vi "GetMultiRobotData.vi"() -> ()   [LabVIEW 2015]
uses:
  <vilib>/robotics/Simulator/NI_Robotics_Simulator.lvlib
  <instrlib>/DC Motor Controller/HAIOL/DC Motor Controller.lvclass
  RobotData.ctl
  <vilib>/robotics/Simulator/Engine/ODESimulator_Engine.lvclass
  <vilib>/robotics/Simulator/Robot Classes/Base/ODESimulator_Base_Robot.lvclass
  <vilib>/robotics/Simulator/Robot Factory/Sensor/Base/ODESimulator_Base_Sensor.lvclass
  <instrlib>/DC Motor Controller/HAIOL/Simulator/DC Motor Controller Simulator.lvclass
  <vilib>/robotics/Simulator/Engine/ctl/DeviceID.ctl
  <vilib>/robotics/Simulator/Robot Factory/Motor/ODESimulator_Motor.lvclass
  SensorType.ctl
panel:
  out "Distance":i32
  out "BUmpsize(s)":i32
  out "Array":T1[](array[typedef])
  out "SensorType":T2 items=["BumperSensor"=1, "DistanceSensor"=2, "AccelerometerSensor"=3, "Wall Sensor"=4, "Unknown"=0]
  in  "manifest file":path
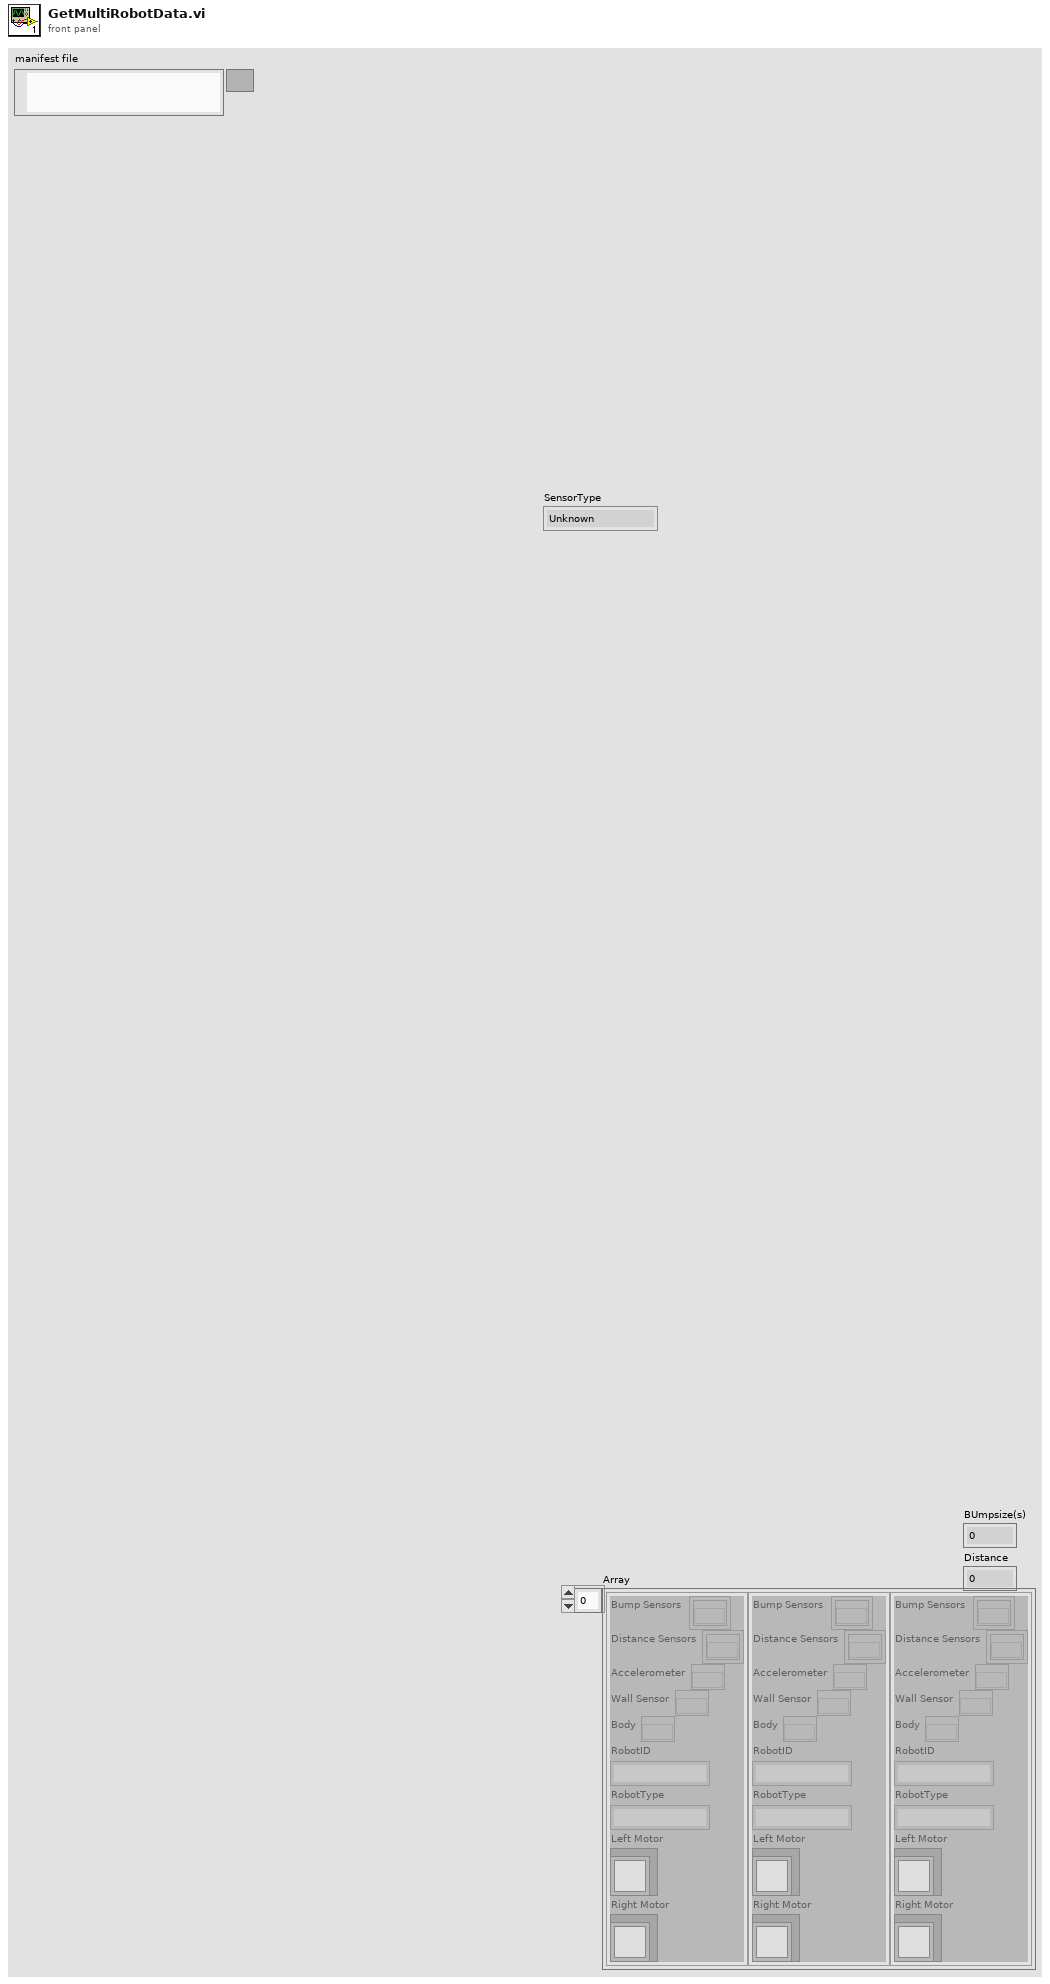
[diagram p1: front panel]
types:
  T1 = typedef "RobotData.ctl" = cluster{"Bump Sensors":refnum<k20>[], "Distance Sensors":refnum<k20>[], "Accelerometer":refnum<k20>, "Wall Sensor":refnum<k20>, "Body":refnum<k20>, "RobotID":string, "RobotType":string, "Left Motor":refnum<class "DC Motor Controller.lvclass">, "Right Motor":refnum<class "DC Motor Controller.lvclass">}
  T2 = typedef "SensorType.ctl" = u16
  T3 = typedef "RobotData.ctl" = cluster{"Bump Sensors":refnum<k20>[], "Distance Sensors":refnum<k20>[], "Accelerometer":refnum<k20>, "Wall Sensor":refnum<k20>, "Body":refnum<k20>, "RobotID":string, "Left Motor":refnum<class "DC Motor Controller.lvclass">, "Right Motor":refnum<class "DC Motor Controller.lvclass">}
  T4 = typedef "NI_Robotics_Simulator.lvlib/DeviceID.ctl" = cluster{"robot ID":string, "sensor/actuator ID":string}
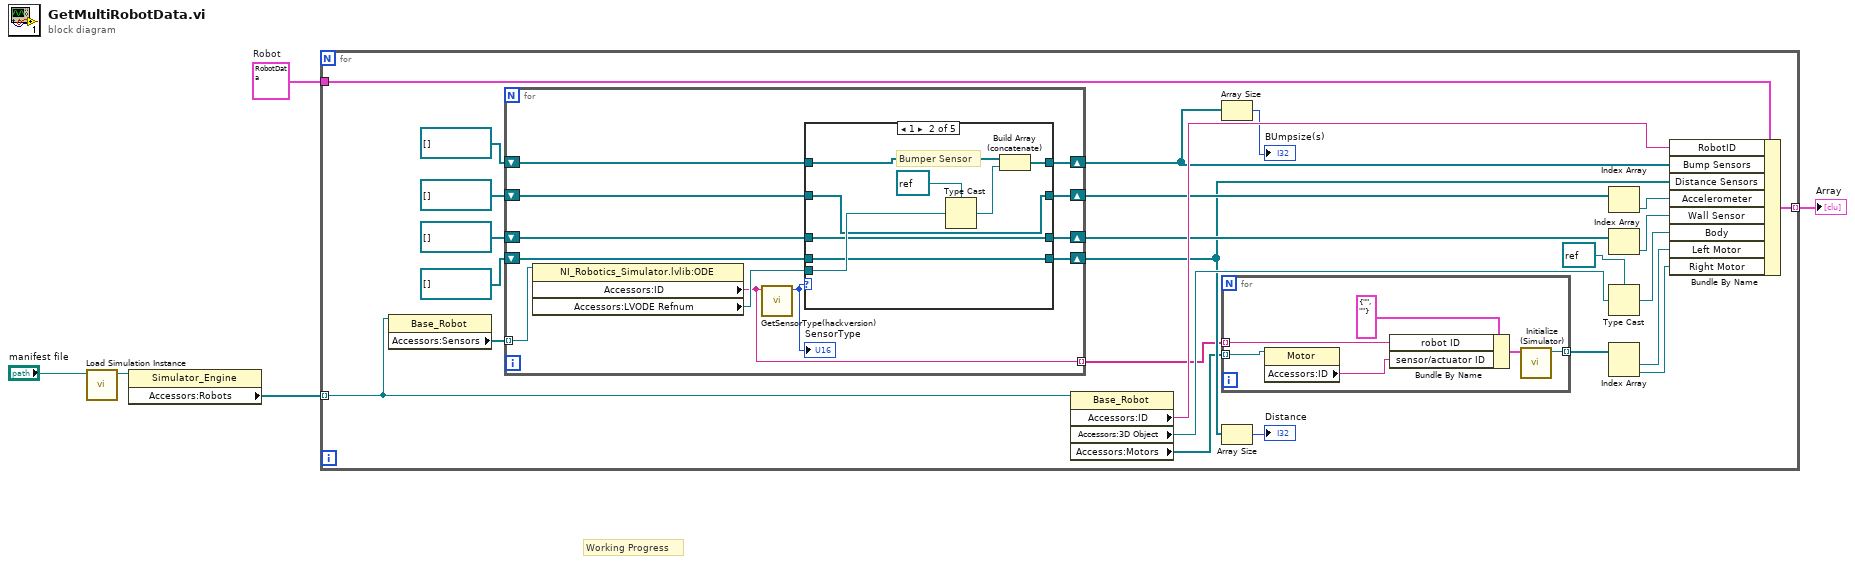
[diagram p0: block diagram]
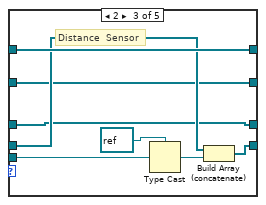
[diagram p3: hidden frame]
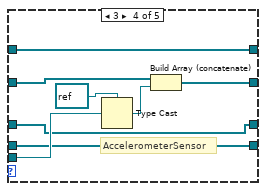
[diagram p4: hidden frame]
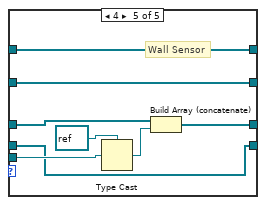
[diagram p5: hidden frame]
diagram:
  w2 = T3 {"Bump Sensors"=[], "Distance Sensors"=[], "Accelerometer"=refnum, "Wall Sensor"=refnum, "Body"=refnum, "RobotID"="", "Left Motor"=refnum, "Right Motor"=refnum}  # Robot
  # "Working Progress"
  n1 = call <vilib>:"Load Simulation Instance.vi"("manifest file"="manifest file") -> ("simulation instance"=w4:refnum<class "ODESimulator_Engine.lvclass">)  [unwired: 9 in, 1 out]
  n2 = property class="Simulator_Engine"(reference=w4) -> ("Accessors:Robots"=w3:refnum<class "ODESimulator_Base_Robot.lvclass">[])  [unwired: 1 in, 2 out]
  n3 = for {
    tunnel: w3 -> [w30] mode=indexing
    tunnel: w2 -> [w28]
    tunnel: [w15] -> w1 mode=indexing
    n4 = property class="Base_Robot"(reference=w30) -> ("Accessors:Sensors"=w29:refnum<class "ODESimulator_Base_Sensor.lvclass">[])  [unwired: 1 in, 2 out]
    n5 = for {
      tunnel: w29 -> [w48] mode=indexing
      shift-right: [w44] -> w14
      shift-left: refnum<k20>[] [] ("Bump Sensors") -> [w45]
      shift-right: [w42] -> w12
      shift-left: refnum<k20>[] [] ("Distance Sensors") -> [w43]
      shift-right: [w40] -> w22
      shift-left: refnum<k20>[] [] ("Bump Sensors") -> [w41]
      shift-right: [w38] -> w20
      shift-left: refnum<k20>[] [] ("Bump Sensors") -> [w39]
      tunnel: [w37] -> w9 mode=indexing
      n6 = property class="NI_Robotics_Simulator.lvlib:ODE"(reference=w48) -> ("Accessors:ID"=w37:string, "Accessors:LVODE Refnum"=w47:refnum<k20>)  [unwired: 1 in, 2 out]
      n7 = call "GetSensorType(hackversion).vi"("Accessors:ID"=w37) -> ("SensorType"=w46:T2)  [unwired: 9 in, 1 out]
      "SensorType" <- w46
      n8 = case shown="1" w46 {
        tunnel: w47 -> [_ w59 w67 w75 w83]
        tunnel: [w52 w57 w65 w74 w82] -> w44
        tunnel: w45 -> [w52 w56 w65 w74 w82]
        tunnel: [w51 w55 w66 w73 w81] -> w42
        tunnel: w43 -> [w51 w55 w64 w73 w81]
        tunnel: [w50 w54 w62 w70 w77] -> w40
        tunnel: w41 -> [w50 w54 w62 w72 w77]
        tunnel: w39 -> [w49 w53 w61 w69 w79]
        tunnel: [w49 w53 w61 w69 w78] -> w38
        frame 0, Default {
        }
        frame 1 {
          # "Bumper Sensor"
          n9 = Type Cast(type=refnum<k20> refnum ("LVODE Refnum"), x=w59) -> (*(type *) &x=w58:refnum<k20>)
          n10 = Build Array (concatenate)(w56, w58) -> (w57:refnum<k20>[])
        }
        frame 2 {
          # "Distance  Sensor"
          n11 = Type Cast(type=refnum<k20> refnum ("LVODE Refnum"), x=w67) -> (*(type *) &x=w63:refnum<k20>)
          n12 = Build Array (concatenate)(w64, w63) -> (w66:refnum<k20>[])
        }
        frame 3 {
          # "AccelerometerSensor"
          n13 = Type Cast(type=refnum<k20> refnum ("LVODE Refnum"), x=w75) -> (*(type *) &x=w71:refnum<k20>)
          n14 = Build Array (concatenate)(w72, w71) -> (w70:refnum<k20>[])
        }
        frame 4 {
          # "Wall Sensor"
          n15 = Type Cast(type=refnum<k20> refnum ("LVODE Refnum"), x=w83) -> (*(type *) &x=w80:refnum<k20>)
          n16 = Build Array (concatenate)(w79, w80) -> (w78:refnum<k20>[])
        }
      }
    }
    n17 = property class="Base_Robot"(reference=w30) -> ("Accessors:ID"=w27:string, "Accessors:3D Object"=w17:refnum<vi>, "Accessors:Motors"=w10:refnum<class "ODESimulator_Motor.lvclass">[])  [unwired: 1 in, 2 out]
    n18 = Array Size(array=w14) -> (size(s)=→"BUmpsize(s)":i32)
    n19 = for {
      tunnel: w10 -> [w34] mode=indexing
      tunnel: w9 -> [w35] mode=indexing
      tunnel: [w31] -> w8 mode=indexing
      n20 = property class="Motor"(reference=w34) -> ("Accessors:ID"=w33:string)  [unwired: 1 in, 2 out]
      n21 = Bundle By Name(cluster=T4 {"robot ID"="", "sensor/actuator ID"=""} ("Device ID"), "robot ID"=w35, "sensor/actuator ID"=w33) -> (w32:T4)
      n22 = call <instrlib>:"Initialize (Simulator).vi"("Device ID"=w32) -> ("DC Motor Controller out"=w31:refnum<class "DC Motor Controller.lvclass">)  [unwired: 9 in, 1 out]
    }
    n23 = Array Size(array=w12) -> (size(s)=→"Distance":i32)
    n24 = Index Array(array=w22) -> (element=w23:refnum<k20>)  [unwired: 1 in]
    n25 = Index Array(array=w20) -> (element=w19:refnum<k20>)  [unwired: 1 in]
    n26 = Type Cast(type=refnum<k20> refnum ("Bump Sensor"), x=w17) -> (*(type *) &x=w16:refnum<k20>)
    n27 = Index Array(array=w8) -> (element #1=w7:refnum<class "DC Motor Controller.lvclass">, element #2=w6:refnum<class "DC Motor Controller.lvclass">)  [unwired: 2 in]
    n28 = Bundle By Name(cluster=w28, "RobotID"=w27, "Bump Sensors"=w14, "Distance Sensors"=w12, "Accelerometer"=w23, "Wall Sensor"=w19, "Body"=w16, "Left Motor"=w7, "Right Motor"=w6) -> (w15:T3)
  }
  "Array" <- w1
